vi "Communication - DBL Data (FGV).vi"(7 "Action":T1=enum."Write", 8 "error in (no error)":errorcluster, 11 "DBL SV":dbl[][](array[numeric])) -> (0 "error out":errorcluster, 3 "DBL SV Out":dbl[][](array[numeric]))   [LabVIEW 2019]
uses:
  Controls/FGV States.ctl
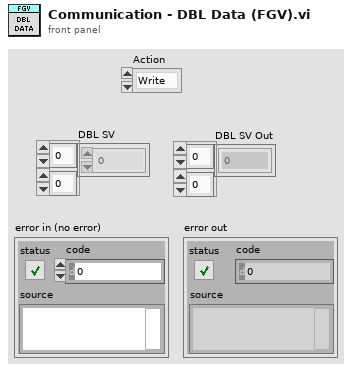
[diagram p1: front panel]
types:
  T1 = typedef "FGV States.ctl" = enum16{"Read", "Write"}
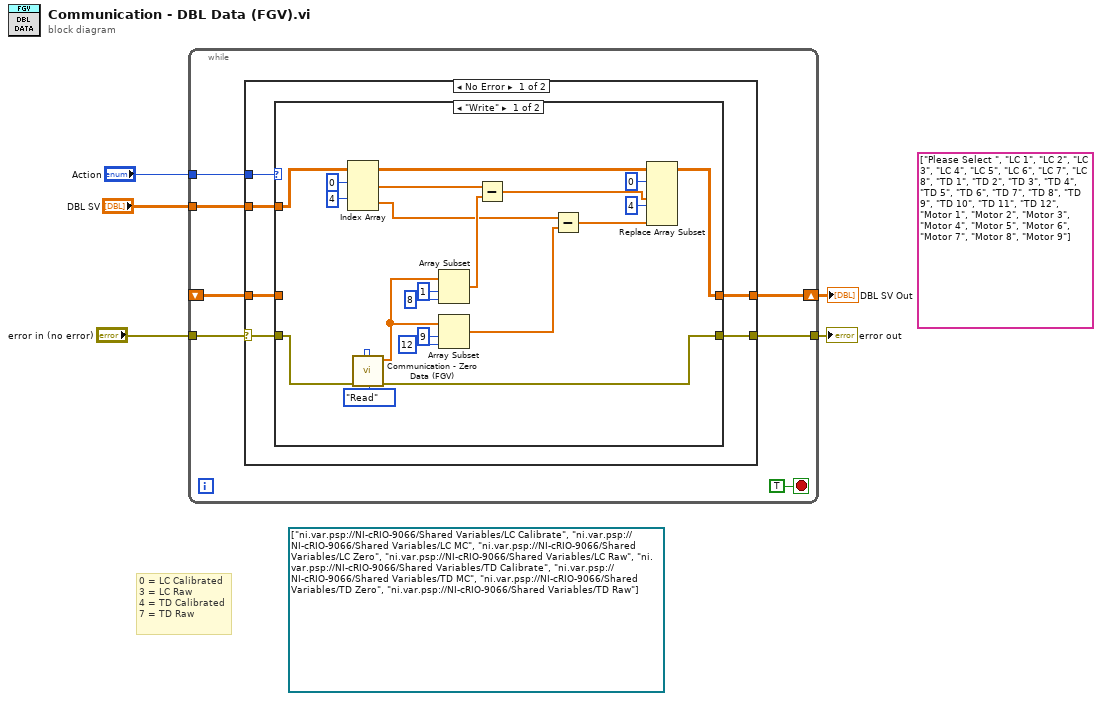
[diagram p0: block diagram]
diagram:
  (unwired) string[] ["Please Select ", "LC 1", "LC 2", "LC 3", "LC 4", "LC 5", "LC 6", "LC 7", "LC 8", "TD 1", "TD 2", "TD 3", "TD 4", "TD 5", "TD 6", "TD 7", "TD 8", "TD 9", "TD 10", "TD 11", "TD 12", "Motor 1", "Motor 2", "Motor 3", "Motor 4", "Motor 5", "Motor 6", "Motor 7", "Motor 8", "Motor 9"] ("string")
  (unwired) refnum<k21>[] ["ni.var.psp://NI-cRIO-9066/Shared Variables/LC Calibrate", "ni.var.psp://NI-cRIO-9066/Shared Variables/LC MC", "ni.var.psp://NI-cRIO-9066/Shared Variables/LC Zero", "ni.var.psp://NI-cRIO-9066/Shared Variables/LC Raw", "ni.var.psp://NI-cRIO-9066/Shared Variables/TD Calibrate", "ni.var.psp://NI-cRIO-9066/Shared Variables/TD MC", "ni.var.psp://NI-cRIO-9066/Shared Variables/TD Zero", "ni.var.psp://NI-cRIO-9066/Shared Variables/TD Raw"]
  # "0 = LC Calibrated\n3 = LC Raw\n4 = TD Calibrated\n7 = TD Raw"
  n1 = while {
    tunnel: "Action" -> [w12]
    tunnel: "DBL SV" -> [w10]
    shift-right: [w11] -> w3
    shift-left: _ -> [w9]
    tunnel: "error in (no error)" -> [w7]
    tunnel: [w6] -> w1
    stop <- TRUE stop-if-true
    n2 = case shown="No Error" w7 {
      selector: w7 -> [w13 w41]
      tunnel: w12 -> [w18 _]
      tunnel: [w17 w42] -> w11
      tunnel: w10 -> [w16 _]
      tunnel: w9 -> [w15 w42]
      tunnel: [w14 w41] -> w6
      frame No Error {
        n3 = case shown="\"Write\"" w18 {
          tunnel: [w26 w39] -> w17
          tunnel: w16 -> [w19 _]
          tunnel: w15 -> [_ w39]
          tunnel: [w27 w40] -> w14
          tunnel: w13 -> [w28 w40]
          frame "Write" {
            n4 = Index Array(array=w19, index (row) #1=0 ("index (row)"), index (row) #2=4 ("index (row)")) -> (element #1=w25:dbl[], element #2=w23:dbl[])  [unwired: 2 in]
            n5 = call "Communication - Zero Data (FGV).vi"("Action"=FGV_States."Read", "error in (no error)"=w28) -> ("error out"=w27:errorcluster, "Zero Out"=w34:dbl[])  [unwired: 8 in]
            n6 = Array Subset(array=w34, index=1, length=8) -> (w24:dbl[])
            n7 = Array Subset(array=w34, index=9, length=12) -> (w22:dbl[])
            n8 = Subtract(x=w25, y=w24) -> (x-y=w20:dbl[])
            n9 = Subtract(x=w23, y=w22) -> (x-y=w21:dbl[])
            n10 = Replace Array Subset(array=w19, new element #1=w20, index (row) #1=0 ("index (row)"), new element #2=w21, index (row) #2=4 ("index (row)")) -> (w26:dbl[][])  [unwired: 2 in]
          }
          frame "Read", Default {
          }
        }
      }
      frame Error {
      }
    }
  }
  "DBL SV Out" <- w3
  "error out" <- w1
